vi "Recognize correct target.vi"(9 "# rectangles":i32, 10 "Rectangles (Calibrated)":T2(array[cluster]), 11 "Image":T3) -> (3 "Image Out":T3)   [LabVIEW 2018]
uses:
  <vilib>/vision/Image Controls.llb/IMAQ Image.ctl
  Dashboard globals.vi
  <vilib>/ptbypt/NI_PtbyPt.lvlib
panel:
  out "Desired Target":T1(radio)=enum."Left End"
  in  "Clamp Points":T4
  in  "Edge detector results":T5
  # "Side of Ship"
  # "End of Ship"
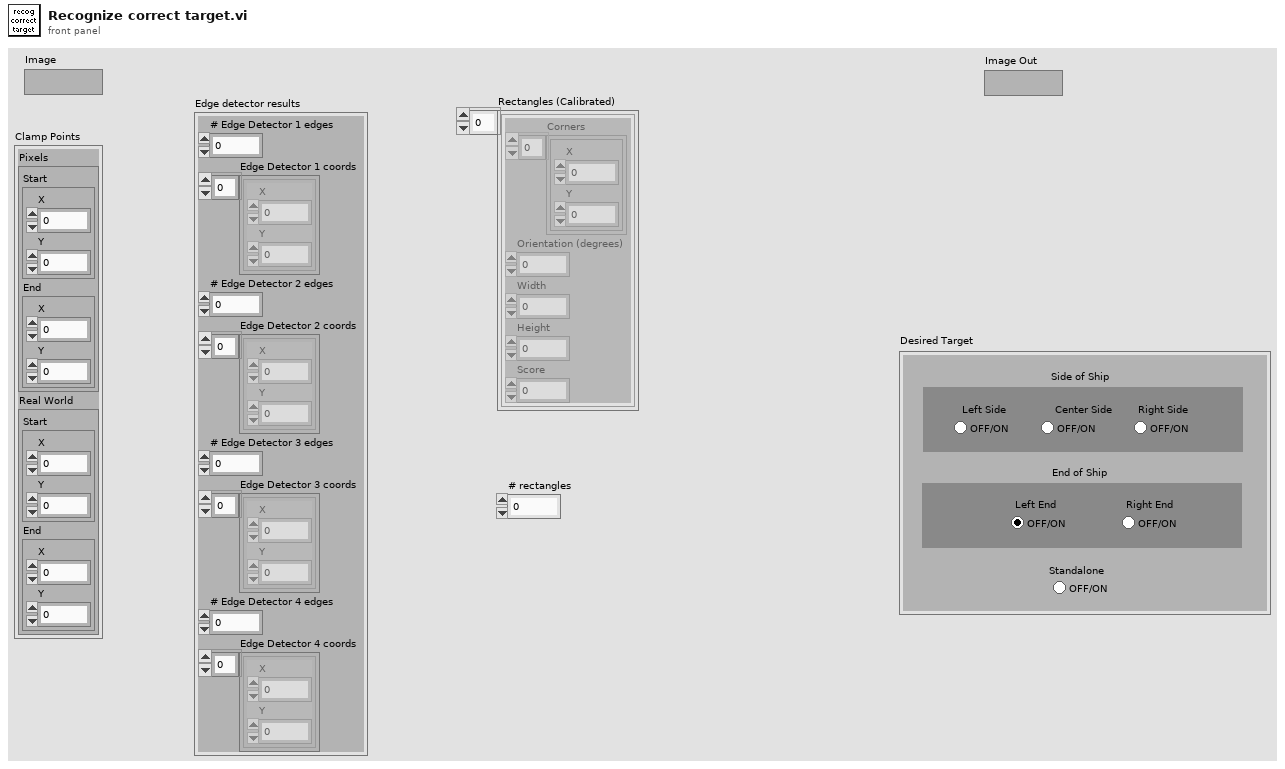
[diagram p1: front panel]
types:
  T1 = enum32{"Left Side", "Center Side", "Right Side", "Left End", "Right End", "Standalone"}
  T2 = cluster{"Corners":cluster{"X":sgl, "Y":sgl}[], "Orientation (degrees)":dbl, "Width":dbl, "Height":dbl, "Score":dbl}[]
  T3 = typedef "IMAQ Image.ctl" = refnum<image>
  T4 = cluster{"Pixels ":cluster{"Start":cluster{"X":dbl, "Y":dbl}, "End":cluster{"X":dbl, "Y":dbl}}, "Real World":cluster{"Start":cluster{"X":dbl, "Y":dbl}, "End":cluster{"X":dbl, "Y":dbl}}}
  T5 = cluster{"# Edge Detector 1 edges":i32, "Edge Detector 1 coords":cluster{"X":sgl, "Y":sgl}[], "# Edge Detector 2 edges":i32, "Edge Detector 2 coords":cluster{"X":sgl, "Y":sgl}[], "# Edge Detector 3 edges":i32, "Edge Detector 3 coords":cluster{"X":sgl, "Y":sgl}[], "# Edge Detector 4 edges":i32, "Edge Detector 4 coords":cluster{"X":sgl, "Y":sgl}[]}
  T6 = cluster{"Start":cluster{"X":dbl, "Y":dbl}, "End":cluster{"X":dbl, "Y":dbl}}
  T7 = enum32{"Ship Side - Left", "Ship Side - Center", "Ship Side - Right", "Ship End - Left", "Ship End - Right", "Rocket or Loading Station"}
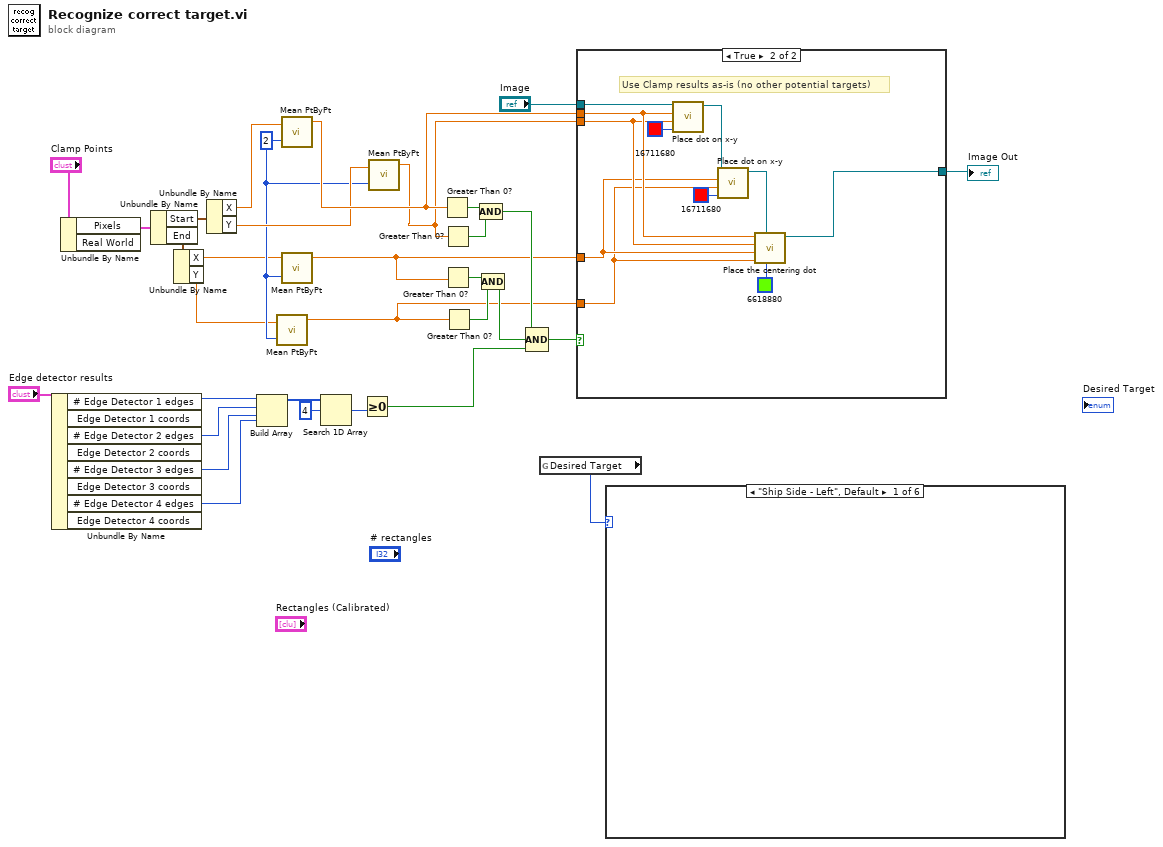
[diagram p0: block diagram]
diagram:
  w14 = 2 ("sample length")
  n1 = Unbundle By Name("Edge detector results") -> ("# Edge Detector 1 edges"=w9:i32, "# Edge Detector 2 edges"=w8:i32, "# Edge Detector 3 edges"=w7:i32, "# Edge Detector 4 edges"=w6:i32)  [unwired: 4 out]
  n2 = Unbundle By Name("Clamp Points") -> ("Pixels"=w27:T6)  [unwired: 1 out]
  n3 = Unbundle By Name(w27) -> ("Start"=w26:cluster{"X":dbl, "Y":dbl}, "End"=w25:cluster{"X":dbl, "Y":dbl})
  n4 = Unbundle By Name(w25) -> ("X"=w11:dbl, "Y"=w13:dbl)
  n5 = Unbundle By Name(w26) -> ("X"=w18:dbl, "Y"=w16:dbl)
  n6 = Build Array(w9, w8, w7, w6) -> (w5:i32[])
  n7 = call <vilib>:"Mean PtByPt.vi"("x"=w13, "sample length"=w14) -> ("mean"=w12:dbl)  [unwired: 2 in, 1 out]
  n8 = call <vilib>:"Mean PtByPt.vi"("x"=w18, "sample length"=w14) -> ("mean"=w17:dbl)  [unwired: 2 in, 1 out]
  n9 = call <vilib>:"Mean PtByPt.vi"("x"=w11, "sample length"=w14) -> ("mean"=w10:dbl)  [unwired: 2 in, 1 out]
  n10 = Search 1D Array(1D array=w5, element=4) -> (index of element=w3:i32)  [unwired: 1 in]
  n11 = Greater Or Equal To 0?(x=w3) -> (x >= 0?=w2:bool)
  n12 = call <vilib>:"Mean PtByPt.vi"("x"=w16, "sample length"=w14) -> ("mean"=w15:dbl)  [unwired: 2 in, 1 out]
  n13 = Greater Than 0?(x=w17) -> (x > 0?=w31:bool)
  n14 = Greater Than 0?(x=w15) -> (x > 0?=w30:bool)
  n15 = Greater Than 0?(x=w10) -> (x > 0?=w28:bool)
  n16 = Greater Than 0?(x=w12) -> (x > 0?=w29:bool)
  n17 = Compound Arithmetic op=AND(w31, w30) -> (w23:bool)
  n18 = Compound Arithmetic op=AND(w28, w29) -> (w22:bool)
  n19 = Compound Arithmetic op=AND(w23, w22, w2) -> (w21:bool)
  n20 = global read "Dashboard globals.vi" "Desired Target"() -> (w1:T7)
  n21 = case shown="True" w21 {
    tunnel: "Image" -> [w33 w44]
    tunnel: w17 -> [_ w38]
    tunnel: w15 -> [_ w37]
    tunnel: w10 -> [_ w36]
    tunnel: w12 -> [_ w35]
    tunnel: [w33 w34] -> w19
    frame False {
    }
    frame True {
      # "Use Clamp results as-is (no other potential targets)"
      n22 = call "Place dot on x-y.vi"("Color"=u32 16711680, "y"=w37, "x"=w38, "Image IN"=w44) -> ("Image OUT"=w41:T3)  [unwired: 7 in]
      n23 = call "Place dot on x-y.vi"("Color"=u32 16711680, "y"=w35, "x"=w36, "Image IN"=w41) -> ("Image OUT"=w40:T3)  [unwired: 7 in]
      n24 = call "Place the centering dot.vi"("Color"=u32 6618880, "Image IN"=w40, "y (R)"=w35, "x (R)"=w36, "y (L)"=w37, "x (L)"=w38) -> ("Image OUT"=w34:T3)  [unwired: 5 in]
    }
  }
  "Image Out" <- w19
  n25 = case shown="\"Ship Side - Left\", Default" w1 {
    frame "Ship Side - Left", Default {
    }
    frame "Ship Side - Center" {
    }
    frame "Ship Side - Right" {
    }
    frame "Ship End - Left" {
    }
    frame "Ship End - Right" {
    }
    frame "Rocket or Loading Station" {
    }
  }
